vi "FTW-SQLite-ExecuteScript.vi"(0 "SQLite Connection":refnum<data-value>, 5 "SQL Script":string, 11 "error in":errorcluster) -> (4 "SQLite Connection out":refnum<data-value>, 6 "SQL Debug String":string, 15 "error out":errorcluster)   [LabVIEW 2014]
uses:
  core/FTW-SQLite-Core-Structure.ctl
panel:
  # "Inputs"
  # "Outputs"
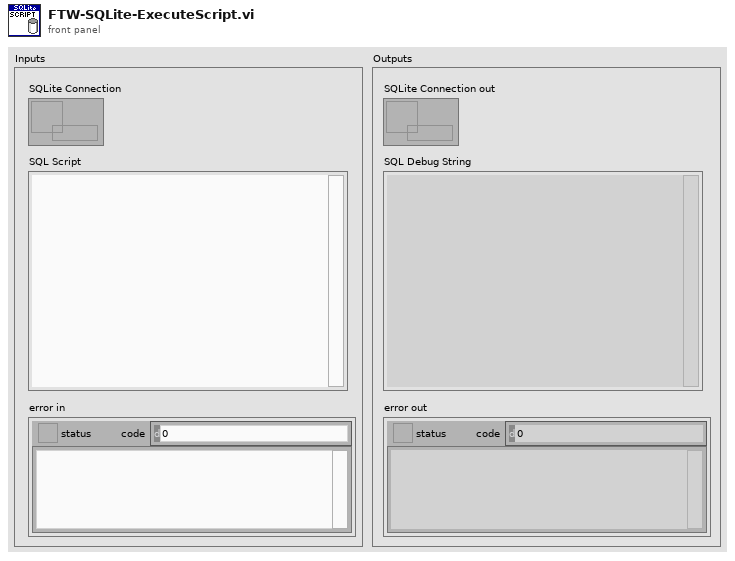
[diagram p1: front panel]
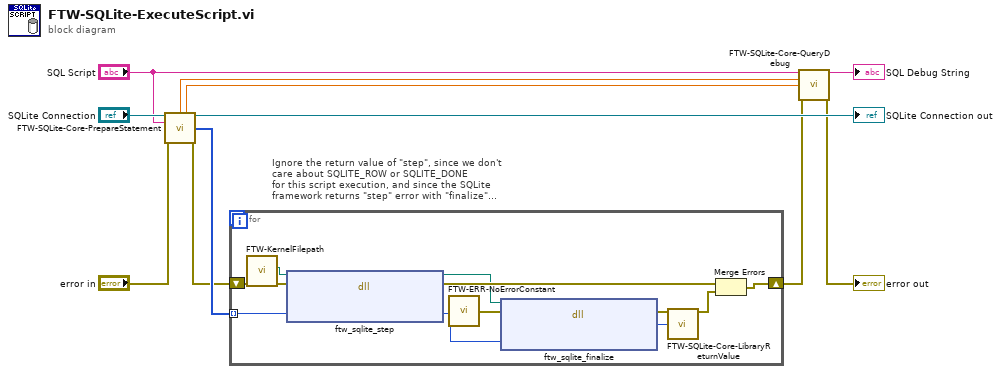
[diagram p0: block diagram]
diagram:
  n1 = call "FTW-SQLite-Core-PrepareStatement.vi"("SQLite Connection"="SQLite Connection", "SQL Statement"="SQL Script", "error in"="error in") -> ("Begin Timestamp"=w2:dbl, "Compile Time"=w1:dbl, "SQLite Connection out"=→"SQLite Connection out":refnum<data-value>, "Prepared Statements"=w9:i64[], "error out"=w8:errorcluster)  [unwired: 8 in]
  n2 = for "Ignore the return value of \"step\", since we don't care about SQLITE_ROW or SQLITE_DONE\nfor this script execution, and since the SQLite framework returns \"step\" error with \"finalize\"\nanyway. Also, we \"finalize\" every prepared statement unconditionally of upstream errors,\nbut only execute \"step\" if no upstream errors." {
    tunnel: w9 -> [w23] mode=indexing
    shift-right: [w18] -> w6
    shift-left: w8 -> [w14]
    n3 = call "FTW-KernelFilepath.vi"("error in"=w14) -> ("error out"=w13:errorcluster, "Library Filepath"=w15:path)  [unwired: 8 in, 1 out]
    n4 = dll-call lib="?" fn="ftw_sqlite_step"(path in=w15, error in=w13, "Prepared Statement Pointer"=w23) -> (path out=w12:path, error out=w19:errorcluster, "Prepared Statement Pointer"=w22:i64)  [unwired: 2 in]
    n5 = call "FTW-ERR-NoErrorConstant.vi"() -> ("no error"=w16:errorcluster)
    n6 = dll-call lib="?" fn="ftw_sqlite_finalize"(path in=w12, error in=w16, "Prepared Statement Pointer"=w22) -> (error out=w21:errorcluster, "Return Value"=w20:i32)  [unwired: 2 in, 1 out]
    n7 = call "FTW-SQLite-Core-LibraryReturnValue.vi"("error in"=w21, "Return Value"=w20) -> ("error out"=w17:errorcluster)  [unwired: 13 in]
    n8 = Merge Errors(w19, w17) -> (w18:errorcluster)
  }
  n9 = call "FTW-SQLite-Core-QueryDebug.vi"("SQL Script"="SQL Script", "Begin Timestamp"=w2, "Compile Time"=w1, "error in"=w6) -> ("SQL Debug String"=→"SQL Debug String":string, "error out"=→"error out":errorcluster)  [unwired: 10 in]
